vi "add.vi"(10 "y":i32, 11 "x":i32) -> (3 "x+y":i32)   [LabVIEW 2015]
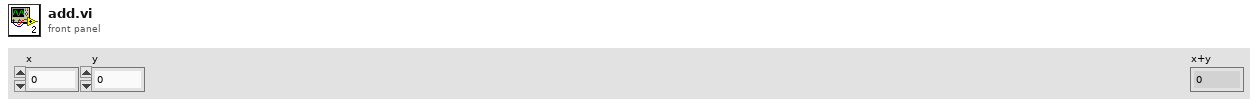
[diagram p1: front panel]
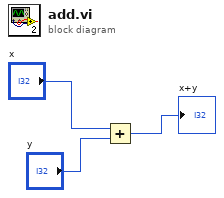
[diagram p0: block diagram]
diagram:
  n1 = Add(x="x", y="y") -> (x+y=→"x+y":i32)
